vi "VerifIdleAsync_01.vi"(8 "error in (no error)":errorcluster, 11 "S4GUI in":refnum<class "S4GUI.lvclass">) -> (0 "error out":errorcluster, 3 "S4GUI out":refnum<class "S4GUI.lvclass">)   [LabVIEW 2018, in "S4GUI.lvclass"]
uses:
  S4GUI.lvclass
  S4GUI.lvclass/S4GUI.ctl
  Acquisition/Acquisition.lvclass
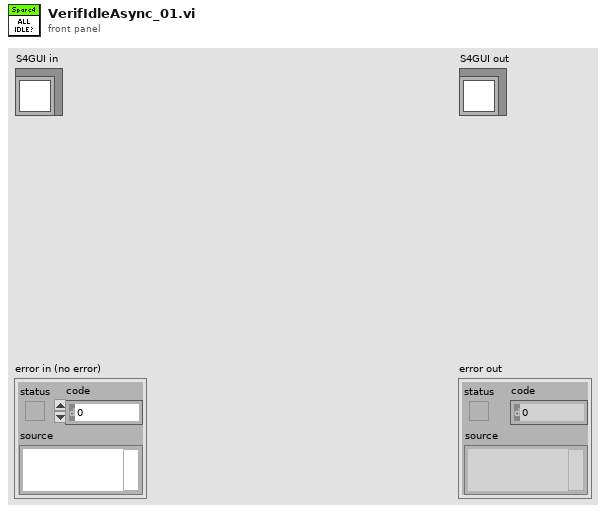
[diagram p1: front panel]
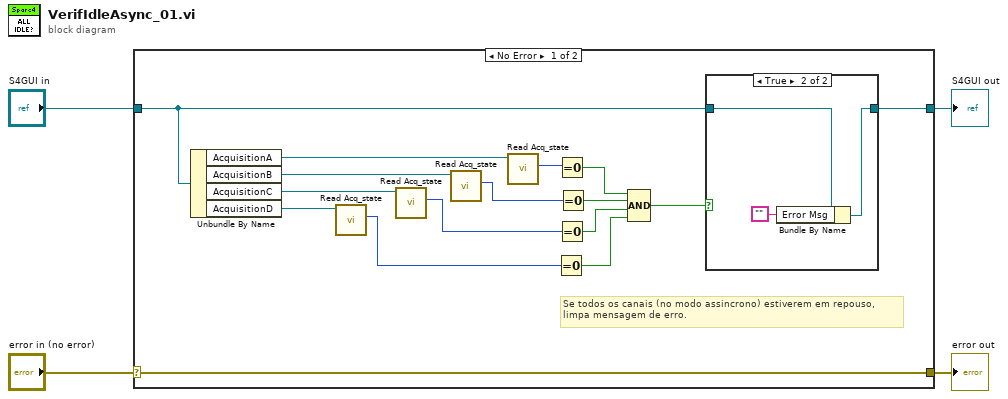
[diagram p0: block diagram]
diagram:
  n1 = case shown="No Error" "error in (no error)" {
    selector: "error in (no error)" -> [w20 w26]
    tunnel: [w20 w26] -> w3
    tunnel: [w5 w25] -> w1
    tunnel: "S4GUI in" -> [w6 w25]
    frame No Error {
      # "Se todos os canais (no modo assincrono) estiverem em repouso,\nlimpa mensagem de erro."
      n2 = Unbundle By Name(w6) -> ("AcquisitionA"=w19:refnum<class "Acquisition.lvclass">, "AcquisitionB"=w18:refnum<class "Acquisition.lvclass">, "AcquisitionC"=w17:refnum<class "Acquisition.lvclass">, "AcquisitionD"=w16:refnum<class "Acquisition.lvclass">)
      n3 = call-dynamic "Read Acq_state.vi"("Acquisition in"=w16) -> ("Acq_state"=w12:u32)  [unwired: 8 in, 2 out]
      n4 = call-dynamic "Read Acq_state.vi"("Acquisition in"=w17) -> ("Acq_state"=w13:u32)  [unwired: 8 in, 2 out]
      n5 = call-dynamic "Read Acq_state.vi"("Acquisition in"=w18) -> ("Acq_state"=w14:u32)  [unwired: 8 in, 2 out]
      n6 = call-dynamic "Read Acq_state.vi"("Acquisition in"=w19) -> ("Acq_state"=w15:u32)  [unwired: 8 in, 2 out]
      n7 = Equal To 0?(x=w12) -> (x = 0?=w8:bool)
      n8 = Equal To 0?(x=w15) -> (x = 0?=w11:bool)
      n9 = Equal To 0?(x=w13) -> (x = 0?=w9:bool)
      n10 = Equal To 0?(x=w14) -> (x = 0?=w10:bool)
      n11 = Compound Arithmetic op=AND(w11, w10, w9, w8) -> (w7:bool)
      n12 = case shown="True" w7 {
        tunnel: w6 -> [w21 w24]
        tunnel: [w21 w23] -> w5
        frame False {
        }
        frame True {
          n13 = Bundle By Name(cluster=w24, "Error Msg"="") -> (w23:refnum<class "S4GUI.lvclass">)
        }
      }
    }
    frame Error {
    }
  }
  "error out" <- w3
  "S4GUI out" <- w1
